vi "Func_Glob_Polysurf_Coeffs_PN.vi"(2 "alpha(rad) coeffs IN":dbl[](array[numeric]), 3 "Ucal coeffs IN":dbl[](array[numeric]), 4 "Action":enum16{"Read", "Write"}(ring)) -> (0 "alpha(rad) coeffs OUT":dbl[](array[numeric]), 1 "Ucal coeffs OUT":dbl[](array[numeric]))   [LabVIEW 2010]
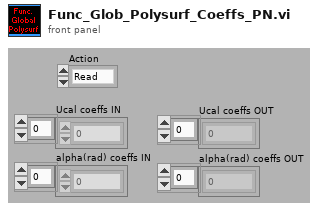
[diagram p1: front panel]
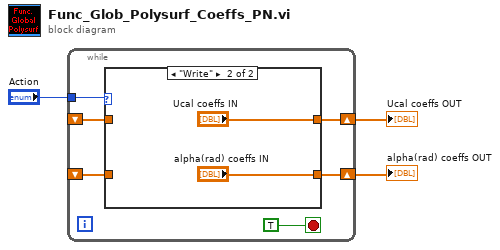
[diagram p0: block diagram]
diagram:
  n1 = while {
    shift-right: [w5] -> w2
    shift-left: _ -> [w7]
    shift-right: [w4] -> w1
    shift-left: _ -> [w6]
    tunnel: "Action" -> [w9]
    stop <- TRUE stop-if-true
    n2 = case shown="\"Write\"" w9 {
      tunnel: w7 -> [w11 _]
      tunnel: w6 -> [w10 _]
      tunnel: [w11 "Ucal coeffs IN"] -> w5
      tunnel: [w10 "alpha(rad) coeffs IN"] -> w4
      frame "Read" {
      }
      frame "Write" {
      }
    }
  }
  "alpha(rad) coeffs OUT" <- w1
  "Ucal coeffs OUT" <- w2
